vi "DoCalibration.vi"() -> ()   [LabVIEW 2015]
uses:
  <vilib>/Utility/file.llb/Read From Spreadsheet File (string).vi
  Desktop/Mari/GlobalData.vi
  <vilib>/Utility/file.llb/Write Delimited Spreadsheet (DBL).vi
panel:
  in  "stop":bool
  out "file path (dialog if empty)":path=path "/home/atlas/Micromegas/ProdData/C_CCD/reference"
  in  "Table (T)/ stiffack(F)":bool
  out "d-param-y-surveyor":dbl=76.253
  out "d-param-x-surveyor":dbl=27.888
  out "cos-phi":dbl=0.99999712
  out "sin-phi":dbl=-0.00239
  out "y-offset":dbl=60.0
  out "x-offset":dbl=24.0
  out "n":dbl
  out "appended array":dbl[][](array[numeric]) format="%.3f"
  out "Array 2":dbl[](array[numeric])
  out "Array":dbl[](array[numeric])
  out "yraw":dbl
  out "xraw":dbl
  out "Misura":string[][](table)
  out "Calib_const":string[][](table)
  out "sinT":dbl
  out "cosT":dbl
  out "ysfera":dbl format="%#.6f"
  out "xsfera":dbl format="%#_8f"
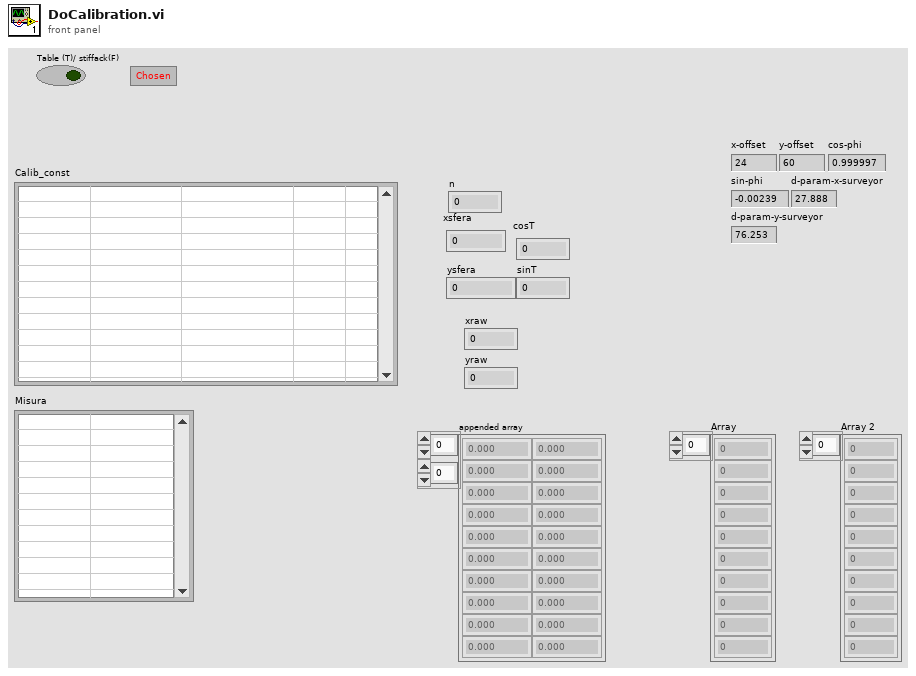
[diagram p1: front panel]
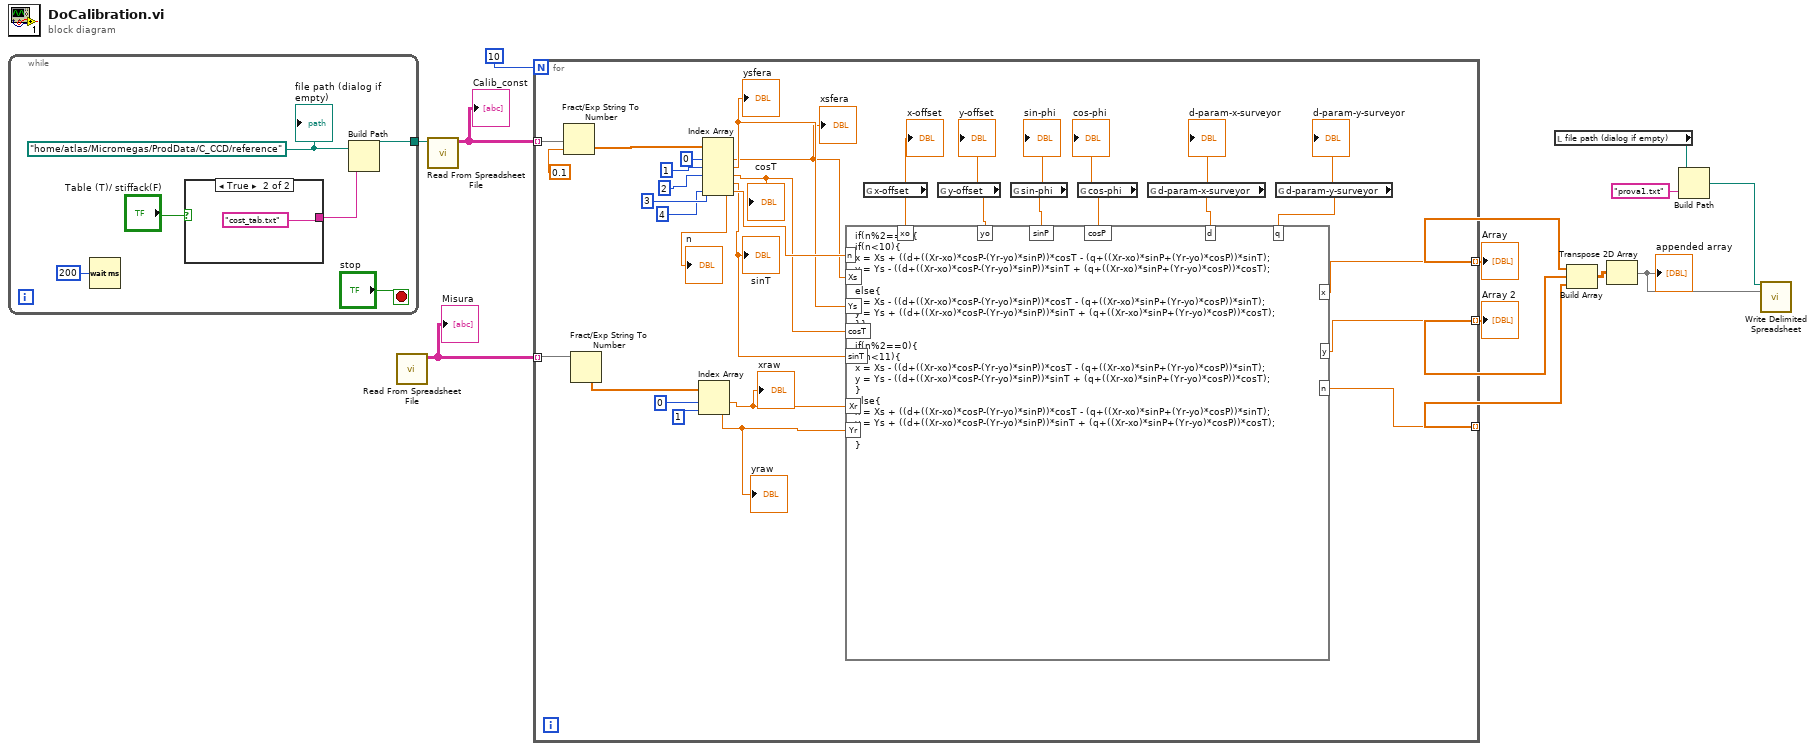
[diagram p0: block diagram]
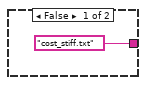
[diagram p2: hidden frame]
diagram:
  n1 = while {
    tunnel: [w18] -> w9
    stop <- "stop" stop-if-true
    w17 = path "/home/atlas/Micromegas/ProdData/C_CCD/reference" ("file path (dialog if empty)")
    n2 = Wait (ms)(milliseconds to wait=u32 200) -> ()  [unwired: 1 out]
    n3 = case shown="True" "Table (T)/ stiffack(F)" {
      tunnel: ["cost_stiff.txt" "cost_tab.txt"] -> w16
      frame False {
      }
      frame True {
      }
    }
    n4 = Build Path(base path=w17, name or relative path=w16) -> (appended path=w18:path)
    "file path (dialog if empty)" <- w17
  }
  n5 = call-poly <vilib>:"Read From Spreadsheet File.vi"() -> ("all rows"=w10:string[][])  [unwired: 7 in, 4 out]
  "Misura" <- w10
  n6 = call-poly <vilib>:"Read From Spreadsheet File.vi"("file path (dialog if empty)"=w9) -> ("all rows"=w11:string[][])  [unwired: 6 in, 4 out]
  "Calib_const" <- w11
  n7 = for {
    N: 10 -> [_]
    tunnel: w11 -> [w44] mode=indexing
    tunnel: w10 -> [w38] mode=indexing
    tunnel: [w37] -> w8 mode=indexing
    tunnel: [w36] -> w7 mode=indexing
    tunnel: [w27] -> w4 mode=indexing
    n8 = Fract/Exp String To Number(string=w44, default (0 dbl)=0.1 ("default (0 DBL)")) -> (number=w43:dbl[])  [unwired: 2 in, 1 out]
    n9 = Fract/Exp String To Number(string=w38) -> (number=w39:dbl[])  [unwired: 3 in, 1 out]
    n10 = Index Array(array=w39, index #1=0 ("index"), index #2=1 ("index")) -> (element #1=w28:dbl, element #2=w32:dbl)
    "xraw" <- w28
    "yraw" <- w32
    n11 = Index Array(array=w43, index #1=0 ("index"), index #2=1 ("index"), index #3=2 ("index"), index #4=3 ("index"), index #5=4 ("index")) -> (element #1=w30:dbl, element #2=w31:dbl, element #3=w33:dbl, element #4=w29:dbl, element #5=w34:dbl)
    "xsfera" <- w30
    "ysfera" <- w31
    "cosT" <- w33
    "sinT" <- w29
    "n" <- w34
    n12 = global read "GlobalData.vi" "x-offset"() -> (w26:dbl)
    "x-offset" <- w26
    n13 = global read "GlobalData.vi" "y-offset"() -> (w25:dbl)
    "y-offset" <- w25
    n14 = global read "GlobalData.vi" "sin-phi"() -> (w24:dbl)
    "sin-phi" <- w24
    n15 = global read "GlobalData.vi" "cos-phi"() -> (w23:dbl)
    "cos-phi" <- w23
    n16 = global read "GlobalData.vi" "d-param-x-surveyor"() -> (w22:dbl)
    "d-param-x-surveyor" <- w22
    n17 = global read "GlobalData.vi" "d-param-y-surveyor"() -> (w21:dbl)
    "d-param-y-surveyor" <- w21
    n18 = formula code="if(n%2==1){\nif(n<10){\nx = Xs + ((d+((Xr-xo)*cosP-(Yr-yo)*sinP))*cosT - (q+((Xr-xo)*sinP+(Yr-yo)*cosP))*sinT);\ny = Ys - ((d+((Xr-xo)*cosP-(Yr-yo)*sinP))*sinT + (q+((Xr-xo)*sinP+(Yr-yo)*cosP))*cosT);\n}\nelse{\nx = Xs - ((d+((Xr-xo)*cosP-(Yr-yo)*sinP))*cosT - (q+((Xr-xo)*sinP+(Yr-yo)*cosP))*sinT);\ny = Ys + ((d+((Xr-xo)*cosP-(Yr-yo)*sinP))*sinT + (q+((Xr-xo)*sinP+(Yr-yo)*cosP))*cosT);\n}}\n\nif(n%2==0){\nif(n<11){\nx = Xs - ((d+((Xr-xo)*cosP-(Yr-yo)*sinP))*cosT - (q+((Xr-xo)*sinP+(Yr-yo)*cosP))*sinT);\ny = Ys - ((d+((Xr-xo)*cosP-(Yr-yo)*sinP))*sinT + (q+((Xr-xo)*sinP+(Yr-yo)*cosP))*cosT);\n}\nelse{\nx = Xs + ((d+((Xr-xo)*cosP-(Yr-yo)*sinP))*cosT - (q+((Xr-xo)*sinP+(Yr-yo)*cosP))*sinT);\ny = Ys + ((d+((Xr-xo)*cosP-(Yr-yo)*sinP))*sinT + (q+((Xr-xo)*sinP+(Yr-yo)*cosP))*cosT);\n}\n}"("Xs"=w30, "sinT"=w29, "Xr"=w28, "Yr"=w32, "cosT"=w33, "Ys"=w31, "xo"=w26, "yo"=w25, "sinP"=w24, "cosP"=w23, "d"=w22, "q"=w21, "n"=w34) -> ("x"=w37:dbl, "y"=w36:dbl, "n"=w27:dbl)
  }
  "Array" <- w8
  "Array 2" <- w7
  n19 = local read "file path (dialog if empty)"() -> (w3:path)
  n20 = Build Array(w8, w7, w4) -> (w6:dbl[][])
  n21 = Transpose 2D Array(2D array=w6) -> (transposed array=w5:dbl[][])
  "appended array" <- w5
  n22 = Build Path(base path=w3, name or relative path="prova1.txt") -> (appended path=w1:path)
  n23 = call-poly <vilib>:"Write Delimited Spreadsheet.vi"("file path (dialog if empty)"=w1, "2D data"=w5) -> ()  [unwired: 12 in, 2 out]
